vi "Teleop.vi"(10 "Match Info":T3={"Autonomous Elapsed Seconds"=0.0, "TeleOp Elapsed Seconds"=0.0, "Disabled Elapsed Seconds"=0.0, "Visited Autonomous"=FALSE, "Visited TeleOp"=FALSE, "Visited Disabled"=FALSE, "Autonomous Settings"={"Autonomous Style"=enum."Independent", "VI Refnum"=refnum}}, 11 "Call Context":T4) -> ()   [LabVIEW 2019]
doc: "This VI is called for each TeleOp packet received from the DS where the robot is not disabled. It is often used to read from the joysticks and update I/O or to update setpoints for timed control loops. It should complete and return within 20 milliseconds or it may miss DS packets."
uses:
  <vilib>/Rock Robotics/WPI/DriverStation/WPI_DriverStationDerivedRobotMode.ctl
  <vilib>/Rock Robotics/WPI/DriverStation/WPI_DriverStationMatch Info.ctl
  numberOfMotors.ctl
  <vilib>/Rock Robotics/WPI/ThirdParty/Phoenix-LabVIEW/Motor Controller/Controls/CTRE_Phoenix_MotorControl_ControlMode.ctl
  <vilib>/Rock Robotics/WPI/Utilities/WPI_GetSetVariantRefNum.vi
  <vilib>/Rock Robotics/Network Tables/NT Write Boolean Array.vi
  <vilib>/Rock Robotics/Network Tables/NT Write Numeric Array.vi
  <vilib>/Rock Robotics/Network Tables/NT Read Boolean.vi
  <vilib>/Rock Robotics/Network Tables/NT Read Number.vi
  <vilib>/Rock Robotics/WPI/ThirdParty/Phoenix-LabVIEW/Motor Controller/Get/CTRE_Phoenix_MotorController_GetSelectedSensorData.vi
panel:
  in  "?":T1(tab)
  in  "motor 3 follows \nmotor 1":enum32{"yes", "no"}(radio)
  in  "motor 2 follows\nmotor 1":enum32{"yes", "no"}(radio)
  in  "Device ID 3":u8
  in  "Device ID 2":u8
  in  "Tertiary motor":enum32{"Talon SRX", "Falcon 500", "Victor SPX"}(radio)
  in  "Secondary motor":enum32{"Talon SRX", "Falcon 500", "Victor SPX"}(radio)
  in  "number of motors":T2
  in  "Primary motor":enum32{"Talon SRX", "Falcon 500"}(radio)
  in  "Apply":bool
  in  "Device ID 1":u8
  in  "intake motor 3 percent output":dbl
  in  "intake motor 2 percent output":dbl
  in  "intake motor 1 percent output":dbl
  out "shooter RPM":dbl
  in  "Shooter Gear Ratio":dbl
  in  "Shooter Percent Output":dbl(slide) scale=-1.0..1.0 scale format="%#_20g"
  out "Shooter RPM":dbl(graph)
  out "Sample Slider 0":dbl(slide) scale=0.0..5.0
  out "Sample Boolean 1":bool
  out "Sample Boolean 0":bool
  # "only works if motor controller has working encoder and shooter gear ratio is non 0"
  # "everything to left is dependant on # of motors"
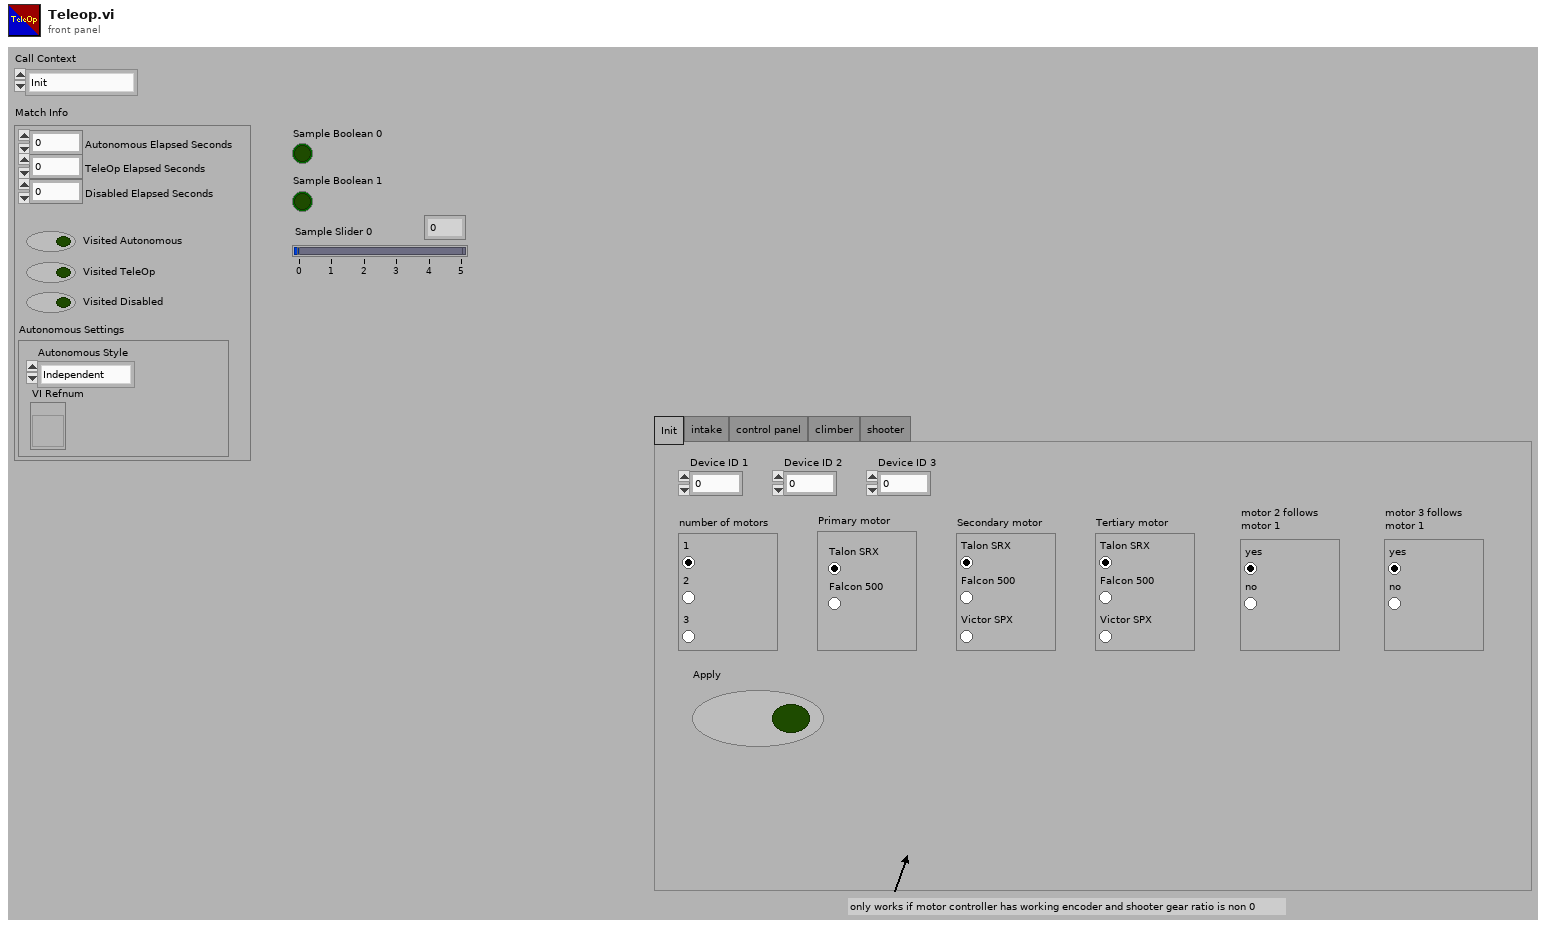
[diagram p1: front panel]
types:
  T1 = enum32{"Init", "intake", "control panel", "climber", "shooter"}
  T2 = typedef "numberOfMotors.ctl" = enum32{"1", "2", "3"}
  T3 = typedef "WPI_DriverStationMatch Info.ctl" = cluster{"Autonomous Elapsed Seconds":dbl, "TeleOp Elapsed Seconds":dbl, "Disabled Elapsed Seconds":dbl, "Visited Autonomous":bool, "Visited TeleOp":bool, "Visited Disabled":bool, "Autonomous Settings":cluster{"Autonomous Style":enum16{"Iterative", "Independent"}, "VI Refnum":refnum<vi>}}
  T4 = typedef "WPI_DriverStationDerivedRobotMode.ctl" = enum16{"Init", "Execute", "Stop"}
  T5 = typedef "WPI_JoystickDevRef.ctl" = cluster{"Device":T6}
  T6 = typedef "WPI_JoystickDeviceEnum.ctl" = enum16{"USB 0", "USB 1", "USB 2", "USB 3", "USB 4", "USB 5"}
  T7 = typedef "WPI_RobotDriveDevRef.ctl" = cluster{"DevStatus":errorcluster, "Motors[]":T8[], "Square Inputs":bool, "Max Output":dbl}
  T8 = typedef "WPI_MotorControlDeviceRef.ctl" = cluster{"DeviceStatus":errorcluster, "Type":T9, "PWM":cluster{"PWM Channel":T10, "DeadBand":T11}, "CAN":cluster{"Device Number":u8, "SetOutput VI Ref":variant, "GetOutput VI Ref":variant, "Enable VI Ref":variant, "Disable VI Ref":variant, "Data":variant}, "Invert":bool, "DIO PWM":cluster{"PWM \"Enable\" Channel":T10, "DIOChannel":T12, "PWM Rate":dbl}}
  T9 = typedef "WPI_MotorControlType.ctl" = enum16{"PWM", "CAN", "DIO PWM"}
  T10 = typedef "FPGA_DIOPWMChannel.ctl" = enum8{"PWM 0", "PWM 1", "PWM 2", "PWM 3", "PWM 4", "PWM 5", "PWM 6", "PWM 7", "PWM 8", "PWM 9", "PWM MXP 0", "PWM MXP 1", "PWM MXP 2", "PWM MXP 3", "PWM MXP 4", "PWM MXP 5", "PWM MXP 6", "PWM MXP 7", "PWM MXP 8", "PWM MXP 9", "Invalid"}
  T11 = typedef "WPI_PWMDeadband.ctl" = cluster{"Name":string, "maxPositivePwm":i32, "minPositivePwm":i32, "centerPwm":i32, "maxNegativePwm":i32, "minNegativePwm":i32, "angularRange":u16}
  T12 = typedef "FPGA_DIOChannel.ctl" = enum8{"DIO 0", "DIO 1", "DIO 2", "DIO 3", "DIO 4", "DIO 5", "DIO 6", "DIO 7", "DIO 8", "DIO 9", "DIO MXP 0", "DIO MXP 1", "DIO MXP 2", "DIO MXP 3", "DIO MXP 4", "DIO MXP 5", "DIO MXP 6", "DIO MXP 7", "DIO MXP 8", "DIO MXP 9", "DIO MXP 10", "DIO MXP 11", "DIO MXP 12", "DIO MXP 13", "DIO MXP 14", "DIO MXP 15", "SPI Port CS1", "SPI Port CS2", "SPI Port CS3", "SPI Port MISO", "SPI Port MOSI", "Invalid"}
  T13 = enum16{"FollowerType_PercentOutput", "FollowerType_AuxOutput1"}
  T14 = typedef "CTRE_Phoenix_MotorControl_ControlMode.ctl" = u16
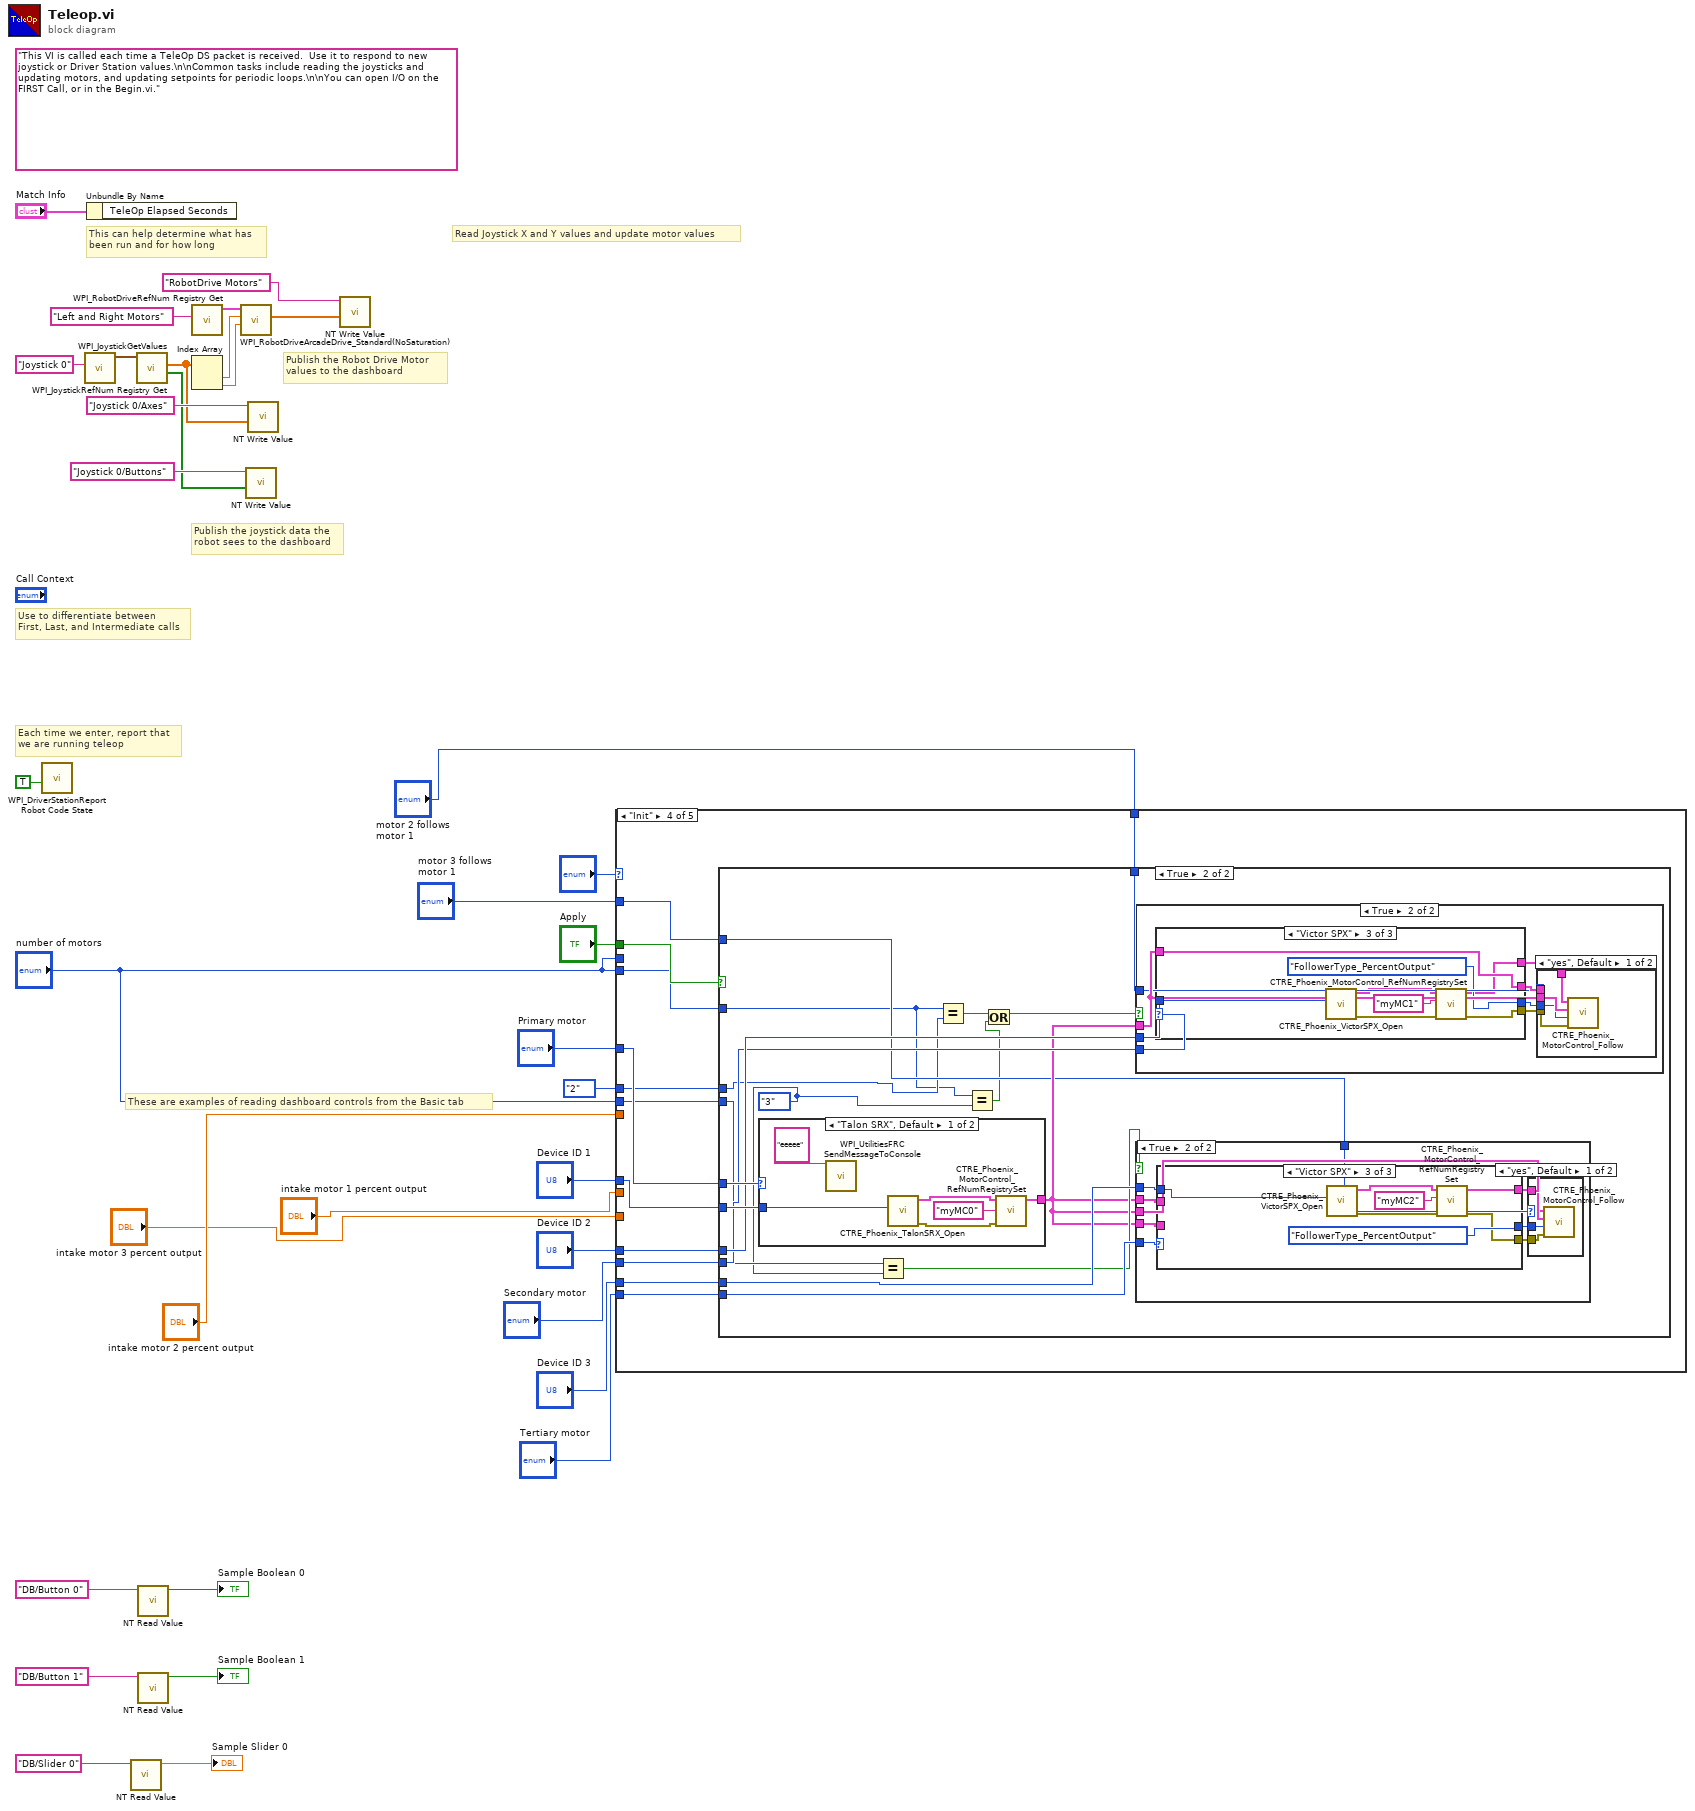
[diagram p0: block diagram]
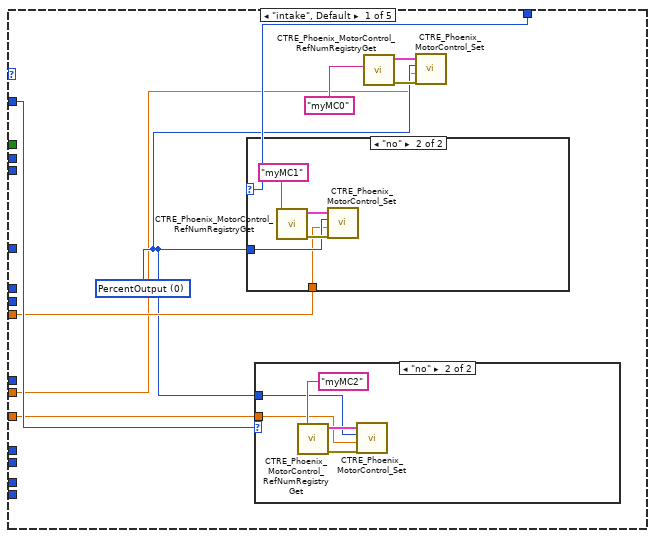
[diagram p2: hidden frame]
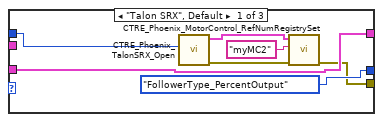
[diagram p11: hidden frame]
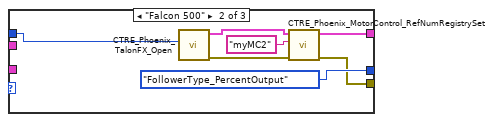
[diagram p12: hidden frame]
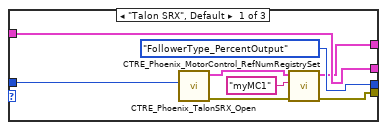
[diagram p15: hidden frame]
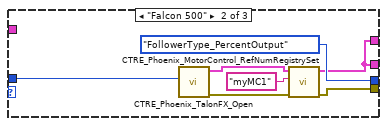
[diagram p16: hidden frame]
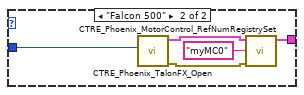
[diagram p17: hidden frame]
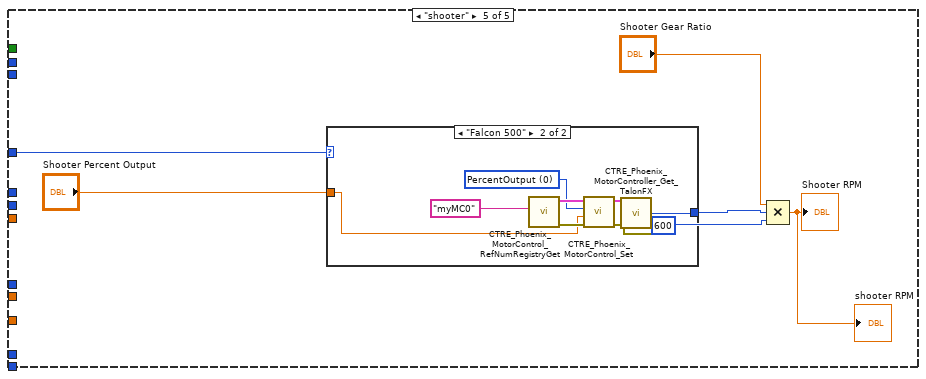
[diagram p18: hidden frame]
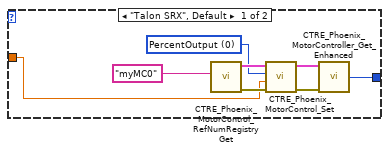
[diagram p19: hidden frame]
diagram:
  (unwired) "This VI is called each time a TeleOp DS packet is received.  Use it to respond to new joystick or Driver Station values.\n\nCommon tasks include reading the joysticks and updating motors, and updating setpoints for periodic loops.\n\nYou can open I/O on the FIRST Call, or in the Begin.vi."
  # "These are examples of reading dashboard controls from the Basic tab"
  # "Publish the Robot Drive Motor\nvalues to the dashboard"
  # "Publish the joystick data the\nrobot sees to the dashboard"
  # "Each time we enter, report that\nwe are running teleop"
  # "Use to differentiate between\nFirst, Last, and Intermediate calls"
  # "This can help determine what has\nbeen run and for how long"
  # "Read Joystick X and Y values and update motor values"
  n1 = call <vilib>:"WPI_DriverStationReport Robot Code State.vi"("TeleOp"=TRUE ("Autonomous")) -> ()  [unwired: 10 in, 1 out]
  n2 = call <vilib>:"WPI_JoystickRefNum Registry Get.vi"("refnum name"="Joystick 0") -> ("JoystickDevRef"=w30:T5)  [unwired: 1 in, 9 out]
  n3 = Unbundle By Name("Match Info") -> ()  [unwired: 1 out]
  n4 = call-poly <vilib>:"NT Read Value.vi"("Name"="DB/Slider 0" ("refnum name")) -> ("Numeric"=→"Sample Slider 0":dbl)  [unwired: 9 in, 1 out]
  n5 = call <vilib>:"WPI_JoystickGetValues.vi"("JoystickDevRef"=w30) -> ("Buttons"=w24:bool[], "Axes"=w25:dbl[])  [unwired: 6 in, 3 out]
  n6 = call-poly <vilib>:"NT Read Value.vi"("Name"="DB/Button 0" ("refnum name")) -> ("Boolean"=→"Sample Boolean 0":bool)  [unwired: 9 in, 1 out]
  n7 = call-poly <vilib>:"NT Read Value.vi"("Name"="DB/Button 1" ("refnum name")) -> ("Boolean"=→"Sample Boolean 1":bool)  [unwired: 9 in, 1 out]
  n8 = call <vilib>:"WPI_RobotDriveRefNum Registry Get.vi"("refnum name"="Left and Right Motors") -> ("RobotDriveDevRef"=w33:T7)  [unwired: 1 in, 9 out]
  n9 = Index Array(array=w25) -> (element #1=w32:dbl, element #2=w28:dbl)  [unwired: 2 in]
  n10 = call <vilib>:"WPI_RobotDriveArcadeDrive_Standard(NoSaturation).vi"("Y axis value"=w28, "X axis value"=w32, "RobotDriveDevRef"=w33) -> ("Motor Values"=w17:dbl[])  [unwired: 1 in, 7 out]
  n11 = call-poly <vilib>:"NT Write Value.vi"("Boolean Array"=w24, "Name"="Joystick 0/Buttons") -> ()  [unwired: 9 in, 1 out]
  n12 = call-poly <vilib>:"NT Write Value.vi"("Numeric Array"=w25, "Name"="Joystick 0/Axes") -> ()  [unwired: 9 in, 1 out]
  n13 = call-poly <vilib>:"NT Write Value.vi"("Numeric Array"=w17, "Name"="RobotDrive Motors") -> ()  [unwired: 9 in, 1 out]
  n14 = case shown="\"Init\"" "?" {
    tunnel: "Apply" -> [_ _ w55 w67 _]
    tunnel: "Primary motor" -> [_ _ _ w66 w170]
    tunnel: "Device ID 1" -> [_ _ _ w65 _]
    tunnel: "Device ID 2" -> [_ _ _ w64 _]
    tunnel: "Secondary motor" -> [_ _ _ w63 _]
    tunnel: "Tertiary motor" -> [_ _ _ w62 _]
    tunnel: "Device ID 3" -> [_ _ _ w61 _]
    tunnel: "number of motors" -> [_ _ _ w60 _]
    tunnel: numberOfMotors."2" ("number of motors") -> [_ _ _ w59 _]
    tunnel: "number of motors" -> [_ _ _ w58 _]
    tunnel: "number of motors" -> [_ _ _ _ _]
    tunnel: "motor 2 follows\nmotor 1" -> [w44 _ _ w57 _]
    tunnel: "motor 3 follows \nmotor 1" -> [w43 _ _ w56 _]
    tunnel: "intake motor 2 percent output" -> [w42 _ _ _ _]
    tunnel: "intake motor 3 percent output" -> [w41 _ _ _ _]
    tunnel: "intake motor 1 percent output" -> [w36 _ _ _ _]
    frame "intake", Default {
      w37 = T14 0 items=["PercentOutput"=0, "Position"=1, "Velocity"=2, "Current"=3, "Follower"=5, "MotionProfile"=6, "MotionMagic"=7, "MotionProfileArc"=10, "Disabled"=15] ("Control Mode")
      n15 = case shown="\"no\"" w44 {
        tunnel: w37 -> [_ w51]
        tunnel: w42 -> [_ w50]
        frame "yes", Default {
        }
        frame "no" {
          n16 = call <vilib>:"CTRE_Phoenix_MotorControl_RefNumRegistryGet.vi"("refnum name"="myMC1") -> ("error out"=w53:errorcluster, "PhoenixMotorControlDevRef"=w52:T8)  [unwired: 9 in]
          n17 = call <vilib>:"CTRE_Phoenix_MotorControl_Set.vi"("error in (no error)"=w53, "Output"=w50, "Control Mode"=w51, "PhoenixMotorControlDevRef"=w52) -> ()  [unwired: 6 in, 2 out]
        }
      }
      n18 = case shown="\"no\"" w43 {
        tunnel: w37 -> [_ w46]
        tunnel: w41 -> [_ w45]
        frame "yes", Default {
        }
        frame "no" {
          n19 = call <vilib>:"CTRE_Phoenix_MotorControl_RefNumRegistryGet.vi"("refnum name"="myMC2") -> ("error out"=w48:errorcluster, "PhoenixMotorControlDevRef"=w47:T8)  [unwired: 9 in]
          n20 = call <vilib>:"CTRE_Phoenix_MotorControl_Set.vi"("error in (no error)"=w48, "Output"=w45, "Control Mode"=w46, "PhoenixMotorControlDevRef"=w47) -> ()  [unwired: 6 in, 2 out]
        }
      }
      n21 = call <vilib>:"CTRE_Phoenix_MotorControl_RefNumRegistryGet.vi"("refnum name"="myMC0") -> ("error out"=w40:errorcluster, "PhoenixMotorControlDevRef"=w39:T8)  [unwired: 9 in]
      n22 = call <vilib>:"CTRE_Phoenix_MotorControl_Set.vi"("error in (no error)"=w40, "Output"=w36, "Control Mode"=w37, "PhoenixMotorControlDevRef"=w39) -> ()  [unwired: 6 in, 2 out]
    }
    frame "control panel" {
    }
    frame "climber" {
      n23 = case shown="True" w55 {
        frame False {
        }
        frame True {
        }
      }
    }
    frame "Init" {
      n24 = case shown="True" w67 {
        tunnel: w66 -> [_ w84]
        tunnel: w65 -> [_ w83]
        tunnel: w64 -> [_ w82]
        tunnel: w63 -> [_ w81]
        tunnel: w62 -> [_ w80]
        tunnel: w61 -> [_ w79]
        tunnel: w60 -> [_ w69]
        tunnel: w59 -> [_ w72]
        tunnel: w58 -> [_ w77]
        tunnel: w57 -> [_ w74]
        tunnel: w56 -> [_ w73]
        frame False {
        }
        frame True {
          w70 = numberOfMotors."3" ("number of motors")
          n25 = case shown="\"Talon SRX\", Default" w84 {
            tunnel: w83 -> [w156 w161]
            tunnel: [w155 w160] -> w75
            frame "Talon SRX", Default {
              n26 = call <vilib>:"WPI_UtilitiesFRC SendMessageToConsole.vi"("Message"="eeeee") -> ()  [unwired: 14 in, 1 out]
              n27 = call <vilib>:"CTRE_Phoenix_TalonSRX_Open.vi"("Device Number"=w156) -> ("error out"=w159:errorcluster, "CAN Talon SRX Ref"=w158:T8)  [unwired: 9 in]
              n28 = call <vilib>:"CTRE_Phoenix_MotorControl_RefNumRegistrySet.vi"("error in (no error)"=w159, "refnum name"="myMC0", "PhoenixMotorControlDevRef"=w158) -> ("PhoenixMotorControlDevRef"=w155:T8)  [unwired: 7 in, 1 out]
            }
            frame "Falcon 500" {
              n29 = call <vilib>:"CTRE_Phoenix_TalonFX_Open.vi"("Device Number"=w161) -> ("error out"=w164:errorcluster, "CAN Talon SRX Ref"=w163:T8)  [unwired: 9 in]
              n30 = call <vilib>:"CTRE_Phoenix_MotorControl_RefNumRegistrySet.vi"("error in (no error)"=w164, "refnum name"="myMC0", "PhoenixMotorControlDevRef"=w163) -> ("PhoenixMotorControlDevRef"=w160:T8)  [unwired: 7 in, 1 out]
            }
          }
          n31 = Equal?(x=w77, y=w70) -> (x = y?=w76:bool)
          n32 = Equal?(x=w69, y=w72) -> (x = y?=w78:bool)
          n33 = Equal?(x=w69, y=w70) -> (x = y?=w68:bool)
          n34 = Or(x=w78, y=w68) -> (x .or. y?=w71:bool)
          n35 = case shown="True" w71 {
            tunnel: w82 -> [_ w126]
            tunnel: w81 -> [_ w125]
            tunnel: w75 -> [_ w124]
            tunnel: w74 -> [_ w120]
            frame False {
            }
            frame True {
              n36 = case shown="\"Victor SPX\"" w125 {
                tunnel: w126 -> [w135 w142 w150]
                tunnel: w124 -> [w134 _ w149]
                tunnel: [w132 w141 w147] -> w123
                tunnel: [T13."FollowerType_PercentOutput" ("FollowerType") T13."FollowerType_PercentOutput" ("FollowerType") T13."FollowerType_PercentOutput" ("FollowerType")] -> w122
                tunnel: [w134 w139 w149] -> w121
                tunnel: [w131 w139 w146] -> w119
                frame "Talon SRX", Default {
                  n37 = call <vilib>:"CTRE_Phoenix_TalonSRX_Open.vi"("Device Number"=w135) -> ("error out"=w138:errorcluster, "CAN Talon SRX Ref"=w137:T8)  [unwired: 9 in]
                  n38 = call <vilib>:"CTRE_Phoenix_MotorControl_RefNumRegistrySet.vi"("error in (no error)"=w138, "refnum name"="myMC1", "PhoenixMotorControlDevRef"=w137) -> ("error out"=w132:errorcluster, "PhoenixMotorControlDevRef"=w131:T8)  [unwired: 7 in]
                }
                frame "Falcon 500" {
                  n39 = call <vilib>:"CTRE_Phoenix_TalonFX_Open.vi"("Device Number"=w142) -> ("error out"=w145:errorcluster, "CAN Talon SRX Ref"=w144:T8)  [unwired: 9 in]
                  n40 = call <vilib>:"CTRE_Phoenix_MotorControl_RefNumRegistrySet.vi"("error in (no error)"=w145, "refnum name"="myMC1", "PhoenixMotorControlDevRef"=w144) -> ("error out"=w141:errorcluster, "PhoenixMotorControlDevRef"=w139:T8)  [unwired: 7 in]
                }
                frame "Victor SPX" {
                  n41 = call <vilib>:"CTRE_Phoenix_VictorSPX_Open.vi"("Device Number"=w150) -> ("error out"=w153:errorcluster, "CAN Talon SRX Ref"=w152:T8)  [unwired: 9 in]
                  n42 = call <vilib>:"CTRE_Phoenix_MotorControl_RefNumRegistrySet.vi"("error in (no error)"=w153, "refnum name"="myMC1", "PhoenixMotorControlDevRef"=w152) -> ("error out"=w147:errorcluster, "PhoenixMotorControlDevRef"=w146:T8)  [unwired: 7 in]
                }
              }
              n43 = case shown="\"yes\", Default" w120 {
                tunnel: w124 -> [w130 _]
                tunnel: w123 -> [w129 _]
                tunnel: w122 -> [w128 _]
                tunnel: w121 -> [_ _]
                tunnel: w119 -> [w127 _]
                frame "yes", Default {
                  n44 = call <vilib>:"CTRE_Phoenix_MotorControl_Follow.vi"("error in (no error)"=w129, "FollowerType"=w128, "Master Controller to Follow"=w130, "PhoenixMotorControlDevRef"=w127) -> ()  [unwired: 6 in, 2 out]
                }
                frame "no" {
                }
              }
            }
          }
          n45 = case shown="True" w76 {
            tunnel: w80 -> [_ w93]
            tunnel: w79 -> [_ w92]
            tunnel: w75 -> [_ w91]
            tunnel: w75 -> [_ w90]
            tunnel: w75 -> [_ w88]
            tunnel: w73 -> [_ w85]
            frame False {
            }
            frame True {
              n46 = case shown="\"Victor SPX\"" w93 {
                tunnel: w92 -> [w101 w108 w115]
                tunnel: w91 -> [_ _ _]
                tunnel: w90 -> [w100 _ _]
                tunnel: [T13."FollowerType_PercentOutput" ("FollowerType") T13."FollowerType_PercentOutput" ("FollowerType") T13."FollowerType_PercentOutput" ("FollowerType")] -> w89
                tunnel: [w100 w106 w114] -> w87
                tunnel: [w98 w105 w112] -> w86
                frame "Talon SRX", Default {
                  n47 = call <vilib>:"CTRE_Phoenix_TalonSRX_Open.vi"("Device Number"=w101) -> ("error out"=w104:errorcluster, "CAN Talon SRX Ref"=w103:T8)  [unwired: 9 in]
                  n48 = call <vilib>:"CTRE_Phoenix_MotorControl_RefNumRegistrySet.vi"("error in (no error)"=w104, "refnum name"="myMC2", "PhoenixMotorControlDevRef"=w103) -> ("error out"=w98:errorcluster)  [unwired: 7 in, 1 out]
                }
                frame "Falcon 500" {
                  n49 = call <vilib>:"CTRE_Phoenix_TalonFX_Open.vi"("Device Number"=w108) -> ("error out"=w111:errorcluster, "CAN Talon SRX Ref"=w110:T8)  [unwired: 9 in]
                  n50 = call <vilib>:"CTRE_Phoenix_MotorControl_RefNumRegistrySet.vi"("error in (no error)"=w111, "refnum name"="myMC2", "PhoenixMotorControlDevRef"=w110) -> ("error out"=w105:errorcluster, "PhoenixMotorControlDevRef"=w106:T8)  [unwired: 7 in]
                }
                frame "Victor SPX" {
                  n51 = call <vilib>:"CTRE_Phoenix_VictorSPX_Open.vi"("Device Number"=w115) -> ("error out"=w118:errorcluster, "CAN Talon SRX Ref"=w117:T8)  [unwired: 9 in]
                  n52 = call <vilib>:"CTRE_Phoenix_MotorControl_RefNumRegistrySet.vi"("error in (no error)"=w118, "refnum name"="myMC2", "PhoenixMotorControlDevRef"=w117) -> ("error out"=w112:errorcluster, "PhoenixMotorControlDevRef"=w114:T8)  [unwired: 7 in]
                }
              }
              n53 = case shown="\"yes\", Default" w85 {
                tunnel: w89 -> [w97 _]
                tunnel: w88 -> [w96 _]
                tunnel: w87 -> [w95 _]
                tunnel: w86 -> [w94 _]
                frame "yes", Default {
                  n54 = call <vilib>:"CTRE_Phoenix_MotorControl_Follow.vi"("error in (no error)"=w94, "FollowerType"=w97, "Master Controller to Follow"=w96, "PhoenixMotorControlDevRef"=w95) -> ()  [unwired: 6 in, 2 out]
                }
                frame "no" {
                }
              }
            }
          }
        }
      }
    }
    frame "shooter" {
      n55 = case shown="\"Falcon 500\"" w170 {
        tunnel: "Shooter Percent Output" -> [w174 w182]
        tunnel: [w171 w179] -> w167
        frame "Talon SRX", Default {
          w175 = T14 0 items=["PercentOutput"=0, "Position"=1, "Velocity"=2, "Current"=3, "Follower"=5, "MotionProfile"=6, "MotionMagic"=7, "MotionProfileArc"=10, "Disabled"=15] ("Control Mode")
          n56 = call <vilib>:"CTRE_Phoenix_MotorControl_RefNumRegistryGet.vi"("refnum name"="myMC0") -> ("error out"=w177:errorcluster, "PhoenixMotorControlDevRef"=w176:T8)  [unwired: 9 in]
          n57 = call <vilib>:"CTRE_Phoenix_MotorControl_Set.vi"("error in (no error)"=w177, "Output"=w174, "Control Mode"=w175, "PhoenixMotorControlDevRef"=w176) -> ("error out"=w172:errorcluster, "PhoenixMotorControlDevRef"=w173:T8)  [unwired: 6 in]
          n58 = call-poly <vilib>:"CTRE_Phoenix_MotorController_Get_Enhanced.vi"("PhoenixMotorControlDevRef"=w173, "error in"=w172) -> ("Velocity (Raw Sensor Units per 100 ms)"=w171:i32)  [unwired: 10 in, 3 out]
        }
        frame "Falcon 500" {
          w183 = T14 0 items=["PercentOutput"=0, "Position"=1, "Velocity"=2, "Current"=3, "Follower"=5, "MotionProfile"=6, "MotionMagic"=7, "MotionProfileArc"=10, "Disabled"=15] ("Control Mode")
          n59 = call <vilib>:"CTRE_Phoenix_MotorControl_RefNumRegistryGet.vi"("refnum name"="myMC0") -> ("error out"=w185:errorcluster, "PhoenixMotorControlDevRef"=w184:T8)  [unwired: 9 in]
          n60 = call <vilib>:"CTRE_Phoenix_MotorControl_Set.vi"("error in (no error)"=w185, "Output"=w182, "Control Mode"=w183, "PhoenixMotorControlDevRef"=w184) -> ("error out"=w180:errorcluster, "PhoenixMotorControlDevRef"=w181:T8)  [unwired: 6 in]
          n61 = call-poly <vilib>:"CTRE_Phoenix_MotorController_Get_TalonFX.vi"("PhoenixMotorControlDevRef"=w181, "error in"=w180) -> ("Velocity (Raw Sensor Units per 100 ms)"=w179:i32)  [unwired: 10 in, 3 out]
        }
      }
      n62 = Compound Arithmetic op=MULTIPLY("Shooter Gear Ratio", w167, 600 ("value")) -> (→"Shooter RPM" →"shooter RPM":dbl)
    }
  }
